vi "Configure VIs for Execution.vi"   [LabVIEW 2017]
types:
  T1 = cluster{"Status Message":refnum<data-value>, "Progress":refnum<data-value>, "Stop":refnum<data-value>}
  T2 = enum16{"Share clones between instances", "Preallocate clone for each instance"}
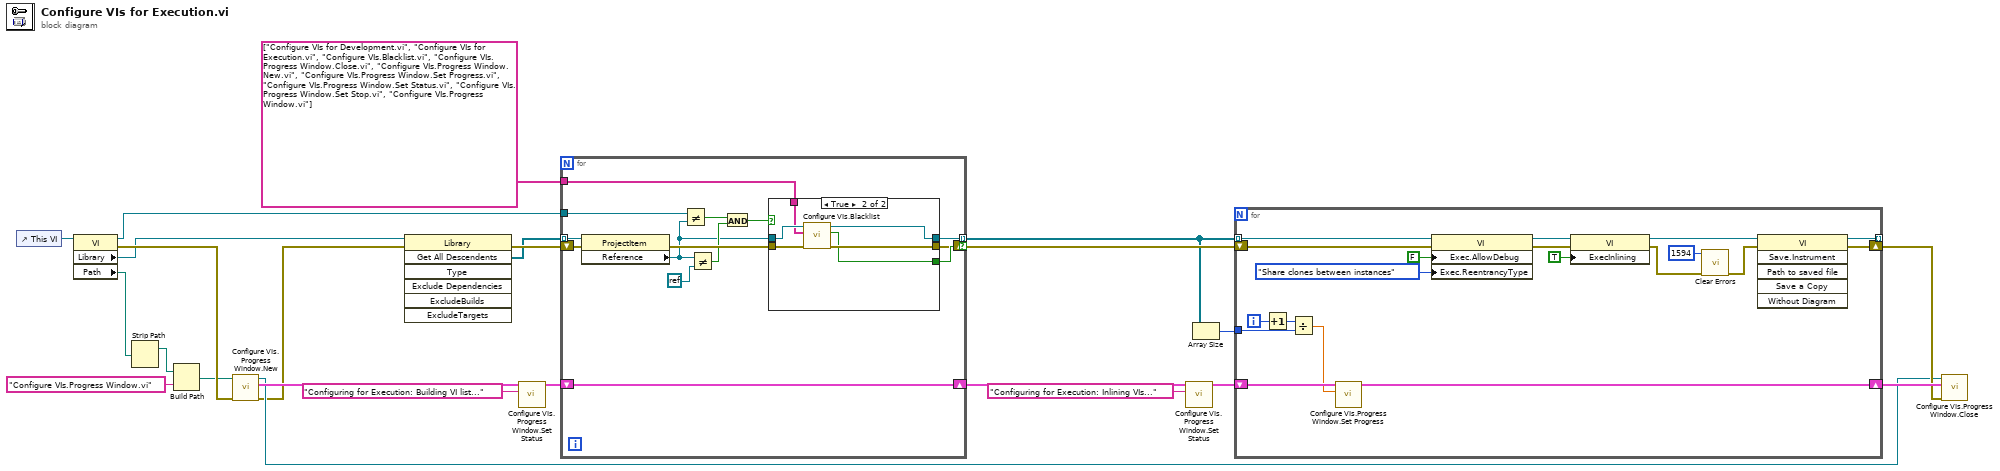
[diagram p0: block diagram]
diagram:
  n1 = control-ref of="This VI"() -> (w23:refnum<vi>)
  n2 = property class="VI"(reference=w23) -> (reference out=w22:refnum<vi>, error out=w24:errorcluster, "Library"=w13:refnum<vi>, "Path"=w2:path)  [unwired: 1 in]
  n3 = Strip Path(path=w2) -> (stripped path=w18:path)  [unwired: 1 out]
  n4 = Build Path(base path=w18, name or relative path="Configure VIs.Progress Window.vi") -> (appended path=w17:path)
  n5 = call "Configure VIs.Progress Window.New.vi"("error in (no error)"=w24, "VI path"=w17) -> ("error out"=w3:errorcluster, "DVRs"=w11:T1, "VI refnum"=w4:refnum<vi>)  [unwired: 7 in]
  n6 = invoke class="Library" method="Get All Descendents"(reference=w13, error in=w3) -> (error out=w20:errorcluster, "All Descendents"=w19:refnum<vi>[])  [unwired: 5 in, 5 out]
  n7 = call "Configure VIs.Progress Window.Set Status.vi"("Status Message"="Configuring for Execution: Building VI list..." ("data value"), "DVRs in"=w11) -> ("DVRs out"=w12:T1)  [unwired: 8 in, 1 out]
  n8 = for {
    tunnel: w19 -> [w38] mode=indexing
    tunnel: [w37] -> w15 mode=indexing if=w36
    tunnel: w22 -> [w34]
    shift-right: [w32] -> w21
    shift-left: w20 -> [w31]
    shift-right: [w26] -> w9
    shift-left: w12 -> [w26]
    tunnel: string[] ["Configure VIs for Development.vi", "Configure VIs for Execution.vi", "Configure VIs.Blacklist.vi", "Configure VIs.Progress Window.Close.vi", "Configure VIs.Progress Window.New.vi", "Configure VIs.Progress Window.Set Progress.vi", "Configure VIs.Progress Window.Set Status.vi", "Configure VIs.Progress Window.Set Stop.vi", "Configure VIs.Progress Window.vi"] ("Blacklist VIs") -> [w25]
    n9 = property class="ProjectItem"(reference=w38, error in=w31) -> (error out=w30:errorcluster, "Reference"=w27:refnum<vi>)  [unwired: 1 out]
    n10 = Not Equal?(x=w34, y=w27) -> (x != y?=w33:bool)
    n11 = Not Equal?(x=w27, y=refnum<k0> refnum) -> (x != y?=w29:bool)
    n12 = And(x=w33, y=w29) -> (x .and. y?=w28:bool)
    n13 = case shown="True" w28 {
      selector: w28 -> [w40 _]
      tunnel: [w41 w45] -> w37
      tunnel: [w40 w43] -> w36
      tunnel: w27 -> [w41 w47]
      tunnel: [w39 w44] -> w32
      tunnel: w30 -> [w39 w46]
      tunnel: w25 -> [_ w42]
      frame False {
      }
      frame True {
        n14 = call "Configure VIs.Blacklist.vi"("error in (no error)"=w46, "Blacklist VIs"=w42, "VI reference in"=w47) -> ("error out"=w44:errorcluster, "valid?"=w43:bool, "VI reference out"=w45:refnum<vi>)  [unwired: 6 in]
      }
    }
  }
  n15 = call "Configure VIs.Progress Window.Set Status.vi"("Status Message"="Configuring for Execution: Inlining VIs..." ("data value"), "DVRs in"=w9) -> ("DVRs out"=w8:T1)  [unwired: 8 in, 1 out]
  n16 = Array Size(array=w15) -> (size(s)=w14:i32)
  n17 = for {
    tunnel: w15 -> [w56] mode=indexing
    tunnel: [w62] -> _ mode=indexing
    shift-right: [w63] -> w5
    shift-left: w21 -> [w55]
    tunnel: w14 -> [w64]
    shift-right: [w59] -> w6
    shift-left: w8 -> [w61]
    i -> [w66]
    n18 = Increment(x=w66) -> (x+1=w65:i32)
    n19 = Divide(x=w65, y=w64) -> (x/y=w60:dbl)
    n20 = call "Configure VIs.Progress Window.Set Progress.vi"("Progress"=w60, "DVRs in"=w61) -> ("DVRs out"=w59:T1)  [unwired: 8 in, 1 out]
    n21 = property class="VI"(reference=w56, error in=w55, "Exec.AllowDebug"=FALSE ("Execution:Allow Debugging"), "Exec.ReentrancyType"=T2."Share clones between instances" ("Execution:Reentrancy Type")) -> (reference out=w50:refnum<vi>, error out=w51:errorcluster)
    n22 = property class="VI"(reference=w50, error in=w51, "ExecInlining"=TRUE ("Execution:Inline SubVI")) -> (reference out=w49:refnum<vi>, error out=w52:errorcluster)
    n23 = call <vilib>:"Clear Errors.vi"("error in (no error)"=w52, "specific error code to clear (0: all)"=1594) -> ("error out"=w48:errorcluster)  [unwired: 4 in, 1 out]
    n24 = invoke class="VI" method="Save.Instrument"(reference=w49, error in=w48) -> (reference out=w62:refnum<vi>, error out=w63:errorcluster)  [unwired: 4 in, 4 out]
  }
  n25 = call "Configure VIs.Progress Window.Close.vi"("error in (no error)"=w5, "DVRs in"=w6, "VI refnum"=w4) -> ()  [unwired: 8 in, 1 out]
